vi "DrivePathToTarget.vi"() -> ()   [LabVIEW 2018]
uses:
  Dawgma Programming Library/Controls/PurePursuit/RobotNeededPathData.ctl
  Framework/Robot Global Data.vi
  Drive/Implementation/Drive Published Globals.vi
panel:
  in  "NoWait":bool
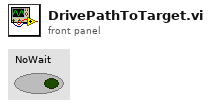
[diagram p1: front panel]
types:
  T1 = typedef "RobotNeededPathData.ctl" = cluster{"Path":cluster{dbl, dbl}[], "MaxVel":dbl, "MaxAccel":dbl, "Backwards?":bool, "PointSpacing":dbl, "LookaheadDist":dbl, "Speed/Curve":dbl, "SlowDistanceAtEnd":dbl, "SlowSpeed":dbl, "MaxDeAccel":dbl}
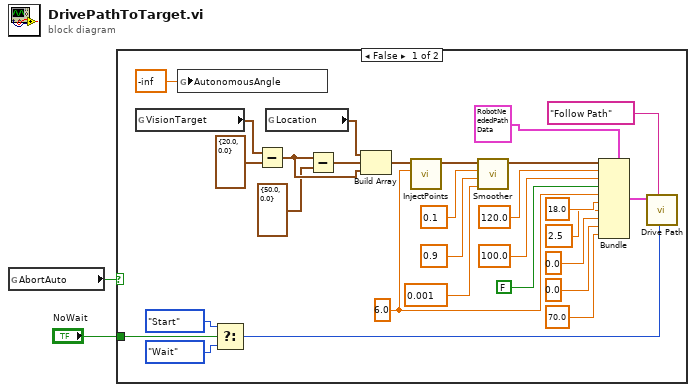
[diagram p0: block diagram]
diagram:
  n1 = global read "Robot Global Data.vi" "AbortAuto"() -> (w2:bool)
  n2 = case shown="False" w2 {
    tunnel: "NoWait" -> [w3 _]
    frame False {
      w17 = 6.0 ("Distance")
      n3 = global read "Robot Global Data.vi" "VisionTarget"() -> (w30:cluster{"X":dbl, "Y":dbl})
      n4 = global write "Robot Global Data.vi" "AutonomousAngle"(-inf ("AutonomousAngle")) -> ()
      n5 = Select(t=enum16{"Start", "Wait"}."Start" ("Synchronication"), s=w3, f=enum16{"Start", "Wait"}."Wait") -> (s? t:f=w4:enum16{"Start", "Wait"})
      n6 = Subtract(x=w30, y=cluster{dbl, dbl} {20.0, 0.0}) -> (x-y=w29:cluster{dbl, dbl})
      n7 = global read "Drive Published Globals.vi" "Location"() -> (w27:cluster{dbl, dbl})
      n8 = Subtract(x=w29, y=cluster{dbl, dbl} {50.0, 0.0}) -> (x-y=w28:cluster{dbl, dbl})
      n9 = Build Array(w27, w28, w29) -> (w7:cluster{dbl, dbl}[])
      n10 = call "InjectPoints.vi"("Spacing"=w17, "Path"=w7) -> ("Path out"=w23:cluster{dbl, dbl}[])  [unwired: 9 in]
      n11 = call "Smoother.vi"("tolerance"=0.001, "B"=0.9, "A"=0.1, "Path"=w23) -> ("SmoothPath"=w24:cluster{dbl, dbl}[])  [unwired: 7 in]
      n12 = Bundle(cluster=T1 {"Path"=[], "MaxVel"=0.0, "MaxAccel"=0.0, "Backwards?"=FALSE, "PointSpacing"=0.0, "LookaheadDist"=0.0, "Speed/Curve"=1.8, "SlowDistanceAtEnd"=12.0, "SlowSpeed"=15.0, "MaxDeAccel"=0.0} ("Path"), "Path"=w24, "MaxVel"=120.0, "MaxAccel"=100.0, "Backwards?"=FALSE, "PointSpacing"=w17, "LookaheadDist"=18.0, "Speed/Curve"=2.5, "SlowDistanceAtEnd"=0.0, "SlowSpeed"=0.0, "MaxDeAccel"=70.0) -> (w22:T1)
      n13 = call "Drive Path.vi"("Synchronication"=w4, "Description"="Follow Path", "Path"=w22) -> ()  [unwired: 8 in, 1 out]
    }
    frame True {
    }
  }
